vi "Next Step.vi"(8 "error in (no error)":errorcluster, 11 "Translation Stage Coarse in":refnum<class "Translation Stage Coarse.lvclass">) -> (0 "error out":errorcluster, 1 "Current Step":u32, 2 "Current Position":dbl, 3 "Translation Stage Coarse out":refnum<class "Translation Stage Coarse.lvclass">)   [LabVIEW 2017, in "Translation Stage Coarse.lvclass"]
doc: "(Dynamic) Move to the next preconfigured step of this Scanner, and return the current position (actual, not intended) of this Scanner. Increment the step counter by one."
uses:
  Translation Stage Coarse.lvclass
  Global/GPIB Numbers.vi
  Scanner/Scanner.lvclass
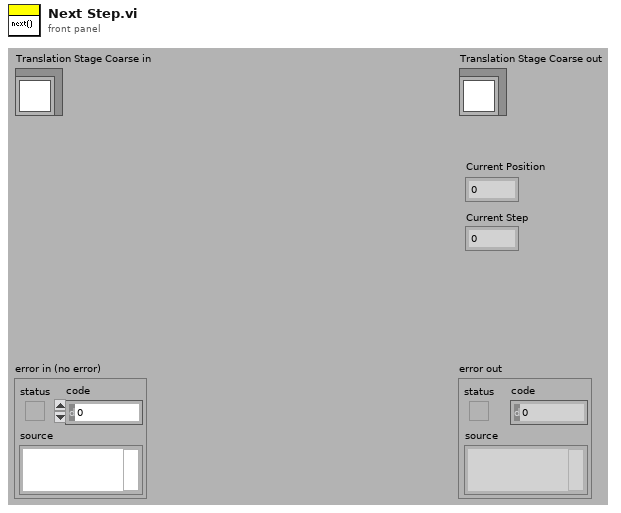
[diagram p1: front panel]
types:
  T1 = typedef "GPIB Type Def.ctl" = cluster{"Name":string, "bus":dbl, "GPIB":dbl, "GPIB as string":string, "byte":i32, "VISA Resource Name":refnum<visa-resource-name>}
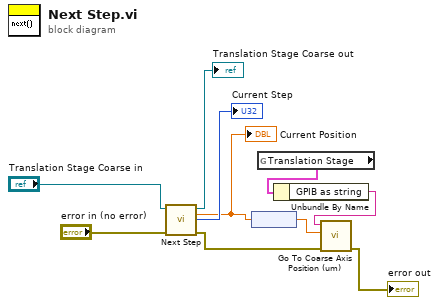
[diagram p0: block diagram]
diagram:
  n1 = call-parent "Next Step.vi"("error in (no error)"="error in (no error)", "Scanner in"="Translation Stage Coarse in") -> ("error out"=w4:errorcluster, "Current Step"=→"Current Step":u32, "Current Position"=w6:dbl, "Scanner out"=→"Translation Stage Coarse out":refnum<class "Translation Stage Coarse.lvclass">)  [unwired: 6 in]
  "Current Position" <- w6
  n2 = node(w6) -> (w5:dbl[unit])
  n3 = global read "GPIB Numbers.vi" "Translation Stage"() -> (w2:T1)
  n4 = Unbundle By Name(w2) -> ("GPIB as string"=w1:string)
  n5 = call "Go To Coarse Axis Position (um).vi"("error in (no error)"=w4, "Coarse Axis Position (um)"=w5, "GPIB # (in): def. 6"=w1) -> ("error out"=→"error out":errorcluster)  [unwired: 7 in, 1 out]
